vi "Write Current Data Offset.vi"(8 "error in (no error)":errorcluster, 10 "Current Data Offset":u16 format="%04x", 11 "1553 SubComponent in":refnum<class "1553 SubComponent.lvclass">) -> (0 "error out":errorcluster, 3 "1553 SubComponent out":refnum<class "1553 SubComponent.lvclass">)   [LabVIEW 2016, in "BCI-1553 API.lvlib" / "1553 SubComponent.lvclass"]
uses:
  1553 SubComponent.lvclass
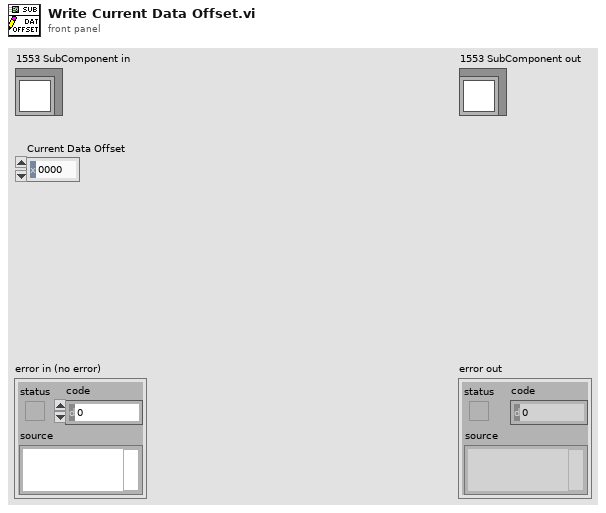
[diagram p1: front panel]
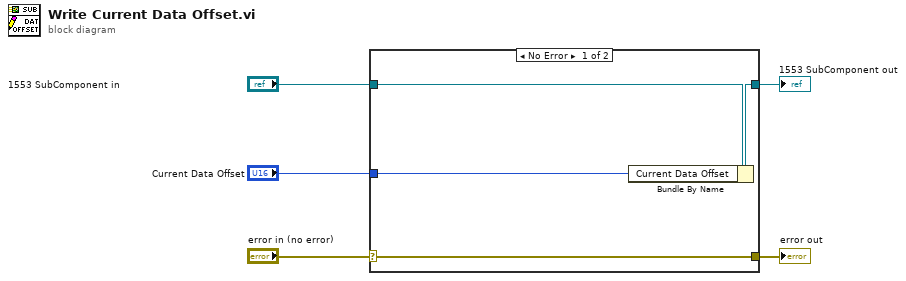
[diagram p0: block diagram]
diagram:
  n1 = case shown="No Error" "error in (no error)" {
    selector: "error in (no error)" -> [w9 w10]
    tunnel: [w9 w10] -> w4
    tunnel: [w7 w11] -> w2
    tunnel: "1553 SubComponent in" -> [w8 w11]
    tunnel: "Current Data Offset" -> [w6 _]
    frame No Error {
      n2 = Bundle By Name(cluster=w8, "Current Data Offset"=w6) -> (w7:refnum<class "1553 SubComponent.lvclass">)
    }
    frame Error {
    }
  }
  "error out" <- w4
  "1553 SubComponent out" <- w2
